vi "S4GUI_001.vi"() -> ()   [LabVIEW 2018] (continued)
                        }
                      }
                    }
                    "Acq status string ch4" <- w721
                    n286 = case shown="True" w726 {
                      tunnel: w729 -> [_ w796]
                      tunnel: w728 -> [_ w799]
                      tunnel: [u32 16739417 w797] -> w727
                      tunnel: ["" ("CamStatus") w796] -> w725
                      frame False {
                      }
                      frame True {
                        n287 = property on="Acq status string ch1" class="Str"() -> ("Text.BGColor"=w798:u32)  [unwired: 2 in, 2 out]
                        n288 = case shown="Default" w796 {
                          tunnel: [w802 u32 13882323 u32 13882323] -> w797
                          tunnel: w799 -> [w801 _ _]
                          tunnel: w798 -> [w800 _ _]
                          frame Default {
                            n289 = case shown="True" w801 {
                              tunnel: [w803 w807] -> w802
                              tunnel: w800 -> [w803 w804]
                              frame False {
                              }
                              frame True {
                                n290 = Equal?(x=w804, y=u32 16776002) -> (x = y?=w806:bool)
                                n291 = case shown="False" w806 {
                                tunnel: [u32 16776002 u32 9346816] -> w807
                                frame False {
                                }
                                frame True {
                                }
                                }
                              }
                            }
                          }
                          frame "IDLE" {
                          }
                          frame "" {
                            # "sem resposta do ACS"
                          }
                        }
                      }
                    }
                    "Acq status string ch1" <- w725
                    n292 = case shown="True" w720 {
                      tunnel: w733 -> [_ w760]
                      tunnel: [u32 16739417 w762] -> w732
                      tunnel: w728 -> [_ w761]
                      tunnel: ["" ("CamStatus") w760] -> w722
                      frame False {
                      }
                      frame True {
                        n293 = property on="Acq status string ch3" class="Str"() -> ("Text.BGColor"=w763:u32)  [unwired: 2 in, 2 out]
                        n294 = case shown="Default" w760 {
                          tunnel: [w766 u32 13882323 u32 13882323] -> w762
                          tunnel: w761 -> [w765 _ _]
                          tunnel: w763 -> [w764 _ _]
                          frame Default {
                            n295 = case shown="True" w765 {
                              tunnel: [w767 w771] -> w766
                              tunnel: w764 -> [w767 w768]
                              frame False {
                              }
                              frame True {
                                n296 = Equal?(x=w768, y=u32 16776002) -> (x = y?=w770:bool)
                                n297 = case shown="True" w770 {
                                tunnel: [u32 16776002 u32 9346816] -> w771
                                frame False {
                                }
                                frame True {
                                }
                                }
                              }
                            }
                          }
                          frame "IDLE" {
                          }
                          frame "" {
                            # "sem resposta do ACS"
                          }
                        }
                      }
                    }
                    "Acq status string ch3" <- w722
                    n298 = case shown="True" w724 {
                      tunnel: w731 -> [_ w778]
                      tunnel: [u32 16739417 w780] -> w730
                      tunnel: w728 -> [_ w779]
                      tunnel: ["" ("CamStatus") w778] -> w723
                      frame False {
                      }
                      frame True {
                        n299 = property on="Acq status string ch2" class="Str"() -> ("Text.BGColor"=w781:u32)  [unwired: 2 in, 2 out]
                        n300 = case shown="\"IDLE\"" w778 {
                          tunnel: [w784 u32 13882323 u32 13882323] -> w780
                          tunnel: w779 -> [w783 _ _]
                          tunnel: w781 -> [w782 _ _]
                          frame Default {
                            n301 = case shown="False" w783 {
                              tunnel: [w785 w789] -> w784
                              tunnel: w782 -> [w785 w786]
                              frame False {
                              }
                              frame True {
                                n302 = Equal?(x=w786, y=u32 16776002) -> (x = y?=w788:bool)
                                n303 = case shown="True" w788 {
                                tunnel: [u32 16776002 u32 9346816] -> w789
                                frame False {
                                }
                                frame True {
                                }
                                }
                              }
                            }
                          }
                          frame "IDLE" {
                          }
                          frame "" {
                            # "sem resposta do ACS"
                          }
                        }
                      }
                    }
                    "Acq status string ch2" <- w723
                    n304 = property on="Acq status string ch2" class="Str"("Text.BGColor"=w730) -> ()  [unwired: 2 in, 2 out]
                    n305 = property on="Acq status string ch1" class="Str"("Text.BGColor"=w727) -> ()  [unwired: 2 in, 2 out]
                    n306 = property on="Acq status string ch3" class="Str"("Text.BGColor"=w732) -> ()  [unwired: 2 in, 2 out]
                    n307 = property on="Acq status string ch4" class="Str"("Text.BGColor"=w735) -> ()  [unwired: 2 in, 2 out]
                  }
                  frame #3 {
                    # "Atualiza status CANAL 1"
                    n308 = Unbundle By Name(w815) -> ("Frames done"=→"Exposure Done ch1":u32, "connection"=→"Channel 1" →"setupCH1":bool, "conf runing"=w812:bool)
                    n309 = property on="setupCH1" class="Bool (strict)"("Blinking"=w812) -> ()  [unwired: 2 in, 2 out]
                  }
                  frame #4 {
                    # "Atualiza status CANAL 2"
                    n310 = Unbundle By Name(w818) -> ("Frames done"=→"Exposure Done ch2":u32, "connection"=→"Channel 2" →"setupCH2":bool, "conf runing"=w816:bool)
                    n311 = property on="setupCH2" class="Bool (strict)"("Blinking"=w816) -> ()  [unwired: 2 in, 2 out]
                  }
                  frame #5 {
                    # "Atualiza status CANAL3"
                    n312 = Unbundle By Name(w822) -> ("Frames done"=→"Exposure Done ch3":u32, "connection"=→"Channel 3" →"setupCH3":bool, "conf runing"=w821:bool)
                    n313 = property on="setupCH3" class="Bool (strict)"("Blinking"=w821) -> ()  [unwired: 2 in, 2 out]
                  }
                  frame #6 {
                    # "Atualiza status CANAL4"
                    n314 = Unbundle By Name(w826) -> ("Frames done"=→"Exposure Done ch4":u32, "connection"=→"Channel 4" →"setupCH4":bool, "conf runing"=w825:bool)
                    n315 = property on="setupCH4" class="Bool (strict)"("Blinking"=w825) -> ()  [unwired: 2 in, 2 out]
                  }
                }
              }
              frame #9 {
                n316 = Unbundle By Name(w829) -> ("Instrument Status.mode"=w828:bool)
                n317 = case shown="True" w828 {
                  tunnel: [0 ("t") w843] -> w830
                  tunnel: w829 -> [_ w832]
                  frame False {
                    # "Fotometria: #PSD = 0"
                  }
                  frame True {
                    # "Polarimetria: calcula #PSD"
                    n318 = Unbundle By Name(w832) -> ("WPROT seq"=w836:u16)
                    n319 = Number To Boolean Array(number=w836) -> (Boolean array=w835:bool[])
                    n320 = for {
                      shift-right: [w847] -> w838
                      shift-left: 0 -> [w845]
                      tunnel: w835 -> [w844] mode=indexing
                      # "calcula qtd de 1s"
                      n321 = Increment(x=w845) -> (x+1=w846:i32)
                      n322 = Select(t=w846, s=w844, f=w845) -> (s? t:f=w847:i32)
                    }
                    n323 = property on="#Polarimetric Sequence Done" class="Slide (strict)"() -> ("Scale.Maximum"=w837:dbl)  [unwired: 2 in, 2 out]
                    n324 = To Long Integer(number=w837) -> (32bit integer=w839:i32)
                    n325 = Subtract(x=w839, y=w838) -> (x-y=w840:i32)
                    n326 = Decrement(x=w840) -> (x-1=w842:i32)
                    n327 = Less Than 0?(x=w842) -> (x < 0?=w841:bool)
                    n328 = Select(t=0, s=w841, f=w842) -> (s? t:f=w843:i32)
                  }
                }
                "#Polarimetric Sequence Done" <- w830
              }
              frame #10 {
                # "OVJ 2022-12-12: \nA visibilidade do Tab ObsEng sempre \nacompanha a habilitação do tab4."
                n329 = Unbundle By Name(w853) -> ("Cluster ExpMode.tab4"=w850:T7, "Cluster Polarimetry"=w874:T15, "Cluster Mode Sync"=w883:T16)
                n330 = case shown="\"Disabled and Grayed Out\"" w850 {
                  tunnel: [TRUE ("Tabs Visible?") w885] -> w852
                  frame "Enabled", Default {
                  }
                  frame "Disabled and Grayed Out" {
                    n331 = disable-structure shown="Enabled" {
                      disable-tunnel: [TRUE ("Tabs Visible?") FALSE ("Tabs Visible?")] -> w885
                      frame Disabled {
                        # "DEBUG"
                      }
                      frame Enabled {
                      }
                    }
                  }
                }
                n332 = property on="Tab ObsEng" class="TabCtl (strict)"("Tabs Visible?"=w852) -> ()  [unwired: 2 in, 2 out]
                n333 = property on="Tab Acq Type" class="TabCtl (strict)"("DisabledEnum"=w850) -> (error out=w851:errorcluster)  [unwired: 2 in, 1 out]
                n334 = Unbundle By Name(w883) -> ("Start SM Text"=w882:string, "Star SM"=w881:T7, "Pause SM"=w880:T7, "Stop SM"=w879:T7, "Abort SM"=w878:T7, "#Cycles"=w877:T7, "SSM"=w876:T7, "Set SM"=w875:T7, "#Index Cycles"=w848:T7)
                n335 = property on="Observer" class="Str"(error in=w851, "DisabledEnum"=w850) -> (error out=w849:errorcluster)  [unwired: 1 in, 1 out]
                n336 = property on="Start SM" class="Bool"("BoolText.Text"=w882) -> ()  [unwired: 2 in, 2 out]
                n337 = property on="set keywords" class="Bool"(error in=w849, "DisabledEnum"=w850) -> ()  [unwired: 1 in, 2 out]
                n338 = property on="#Cycles Done" class="Slide (strict)"("DisabledEnum"=w848) -> ()  [unwired: 2 in, 2 out]
                n339 = property on="Start SM" class="Bool"("DisabledEnum"=w881) -> ()  [unwired: 2 in, 2 out]
                n340 = property on="Stop SM" class="Bool"("DisabledEnum"=w879) -> ()  [unwired: 2 in, 2 out]
                n341 = property on="Abort SM" class="Bool"("DisabledEnum"=w878) -> ()  [unwired: 2 in, 2 out]
                n342 = property on="Pause SM" class="Bool"("DisabledEnum"=w880) -> ()  [unwired: 2 in, 2 out]
                n343 = property on="# Cycles" class="DigNum (strict)"("DisabledEnum"=w877) -> ()  [unwired: 2 in, 2 out]
                n344 = property on="SSM" class="Ring (strict)"("DisabledEnum"=w876) -> ()  [unwired: 2 in, 2 out]
                n345 = property on="Set SM" class="Bool"("DisabledEnum"=w875) -> ()  [unwired: 2 in, 2 out]
                n346 = Unbundle By Name(w874) -> ("Lambda Selector"=w873:T7, "Calibrator Selector"=w872:T7, "Set Waveplate"=w871:T7, "Select Positions"=w870:T7, "P0"=w869:T7, "P8"=w868:T7, "P1"=w867:T7, "P9"=w866:T7, "P2"=w865:T7, "P10"=w864:T7, "P3"=w863:T7, "P11"=w862:T7, "P4"=w861:T7, "P12"=w860:T7, "P5"=w859:T7, "P13"=w858:T7, "P6"=w857:T7, "P14"=w856:T7, "P7"=w855:T7, "P15"=w854:T7)
                n347 = property on="P0" class="Bool (strict)"("DisabledEnum"=w869) -> ()  [unwired: 2 in, 2 out]
                n348 = property on="Lambda Selector" class="Ring (strict)"("DisabledEnum"=w873) -> ()  [unwired: 2 in, 2 out]
                n349 = property on="Calibrator Selector" class="Ring (strict)"("DisabledEnum"=w872) -> ()  [unwired: 2 in, 2 out]
                n350 = property on="Set Waveplate" class="Bool"("DisabledEnum"=w871) -> ()  [unwired: 2 in, 2 out]
                n351 = property on="P1" class="Bool (strict)"("DisabledEnum"=w867) -> ()  [unwired: 2 in, 2 out]
                n352 = property on="P2" class="Bool (strict)"("DisabledEnum"=w865) -> ()  [unwired: 2 in, 2 out]
                n353 = property on="P3" class="Bool (strict)"("DisabledEnum"=w863) -> ()  [unwired: 2 in, 2 out]
                n354 = property on="P4" class="Bool (strict)"("DisabledEnum"=w861) -> ()  [unwired: 2 in, 2 out]
                n355 = property on="P5" class="Bool (strict)"("DisabledEnum"=w859) -> ()  [unwired: 2 in, 2 out]
                n356 = property on="P6" class="Bool (strict)"("DisabledEnum"=w857) -> ()  [unwired: 2 in, 2 out]
                n357 = property on="P7" class="Bool (strict)"("DisabledEnum"=w855) -> ()  [unwired: 2 in, 2 out]
                n358 = property on="Select Positions" class="Ring (strict)"("DisabledEnum"=w870) -> ()  [unwired: 2 in, 2 out]
                n359 = property on="P8" class="Bool (strict)"("DisabledEnum"=w868) -> ()  [unwired: 2 in, 2 out]
                n360 = property on="P15" class="Bool (strict)"("DisabledEnum"=w854) -> ()  [unwired: 2 in, 2 out]
                n361 = property on="P9" class="Bool (strict)"("DisabledEnum"=w866) -> ()  [unwired: 2 in, 2 out]
                n362 = property on="P10" class="Bool (strict)"("DisabledEnum"=w864) -> ()  [unwired: 2 in, 2 out]
                n363 = property on="P11" class="Bool (strict)"("DisabledEnum"=w862) -> ()  [unwired: 2 in, 2 out]
                n364 = property on="P12" class="Bool (strict)"("DisabledEnum"=w860) -> ()  [unwired: 2 in, 2 out]
                n365 = property on="P13" class="Bool (strict)"("DisabledEnum"=w858) -> ()  [unwired: 2 in, 2 out]
                n366 = property on="P14" class="Bool (strict)"("DisabledEnum"=w856) -> ()  [unwired: 2 in, 2 out]
              }
              frame #11 {
                n367 = Unbundle By Name(w902) -> ("Cluster Mode CH1"=w889:T17, "Cluster Mode Sync"=w888:T16)
                n368 = Unbundle By Name(w889) -> ("Start ch1 Text"=w901:string, "#cycles ch1"=w900:T7, "Start ch1"=w899:T7, "Pause ch1"=w898:T7, "Abort ch1"=w897:T7, "Stop ch1"=w896:T7, "Exptime ch1"=w895:T7, "Exp ch1"=w894:T7, "Set Cooler"=w893:T7, "Set Temp"=w892:T7)
                n369 = Unbundle By Name(w888) -> ("#Index Cycles"=w891:T7)
                n370 = case shown="Default" w891 {
                  tunnel: [T7."Enabled" ("#Index Cycles") T7."Disabled and Grayed Out" ("#Index Cycles")] -> w890
                  frame "Disabled and Grayed Out" {
                  }
                  frame Default {
                  }
                }
                n371 = property on="Start ch1" class="Bool"("BoolText.Text"=w901) -> ()  [unwired: 2 in, 2 out]
                n372 = property on="Abort ch1" class="Bool"("DisabledEnum"=w897) -> ()  [unwired: 2 in, 2 out]
                n373 = property on="Stop ch1" class="Bool"("DisabledEnum"=w896) -> ()  [unwired: 2 in, 2 out]
                n374 = property on="#cycles ch1" class="DigNum (strict)"("DisabledEnum"=w900) -> ()  [unwired: 2 in, 2 out]
                n375 = property on="Cooler 1" class="Bool (strict)"("DisabledEnum"=w893) -> ()  [unwired: 2 in, 2 out]
                n376 = property on="Exptime ch1" class="DigNum (strict)"("DisabledEnum"=w895) -> ()  [unwired: 2 in, 2 out]
                n377 = property on="Start ch1" class="Bool"("DisabledEnum"=w899) -> ()  [unwired: 2 in, 2 out]
                n378 = property on="Set Temp 1" class="Bool"("DisabledEnum"=w892) -> ()  [unwired: 2 in, 2 out]
                n379 = property on="Exp ch1" class="DigNum (strict)"("DisabledEnum"=w894) -> ()  [unwired: 2 in, 2 out]
                n380 = property on="Cycles Done ch1" class="Slide (strict)"("DisabledEnum"=w890) -> ()  [unwired: 2 in, 2 out]
                n381 = property on="Pause ch1" class="Bool"("DisabledEnum"=w898) -> ()  [unwired: 2 in, 2 out]
              }
              frame #12 {
                n382 = Unbundle By Name(w919) -> ("Cluster Mode CH2"=w918:T18, "Cluster Mode Sync"=w906:T16)
                n383 = Unbundle By Name(w906) -> ("#Index Cycles"=w907:T7)
                n384 = Unbundle By Name(w918) -> ("Start ch2 Text"=w917:string, "#cycles ch2"=w916:T7, "Start ch2"=w915:T7, "Pause ch2"=w914:T7, "Stop ch2"=w913:T7, "Abort ch2"=w912:T7, "Exptime ch2"=w911:T7, "Exp ch2"=w910:T7, "Set Cooler"=w909:T7, "Set Temp"=w908:T7)
                n385 = case shown="\"Disabled and Grayed Out\"" w907 {
                  tunnel: [T7."Enabled" ("#Index Cycles") T7."Disabled and Grayed Out" ("#Index Cycles")] -> w905
                  frame "Disabled and Grayed Out" {
                  }
                  frame Default {
                  }
                }
                n386 = property on="Start ch2" class="Bool"("BoolText.Text"=w917) -> ()  [unwired: 2 in, 2 out]
                n387 = property on="Stop ch2" class="Bool"("DisabledEnum"=w913) -> ()  [unwired: 2 in, 2 out]
                n388 = property on="Abort ch2" class="Bool"("DisabledEnum"=w912) -> ()  [unwired: 2 in, 2 out]
                n389 = property on="Cooler 2" class="Bool (strict)"("DisabledEnum"=w909) -> ()  [unwired: 2 in, 2 out]
                n390 = property on="#cycles ch2" class="DigNum (strict)"("DisabledEnum"=w916) -> ()  [unwired: 2 in, 2 out]
                n391 = property on="Exptime ch2" class="DigNum (strict)"("DisabledEnum"=w911) -> ()  [unwired: 2 in, 2 out]
                n392 = property on="Set Temp 2" class="Bool"("DisabledEnum"=w908) -> ()  [unwired: 2 in, 2 out]
                n393 = property on="Start ch2" class="Bool"("DisabledEnum"=w915) -> ()  [unwired: 2 in, 2 out]
                n394 = property on="Cycles Done ch2" class="Slide (strict)"("DisabledEnum"=w905) -> ()  [unwired: 2 in, 2 out]
                n395 = property on="Exp ch2" class="DigNum (strict)"("DisabledEnum"=w910) -> ()  [unwired: 2 in, 2 out]
                n396 = property on="Pause ch2" class="Bool"("DisabledEnum"=w914) -> ()  [unwired: 2 in, 2 out]
              }
              frame #13 {
                n397 = Unbundle By Name(w936) -> ("Cluster Mode CH3"=w935:T19, "Cluster Mode Sync"=w923:T16)
                n398 = Unbundle By Name(w923) -> ("#Index Cycles"=w924:T7)
                n399 = Unbundle By Name(w935) -> ("Start ch3 Text"=w934:string, "#cycles ch3"=w933:T7, "Start ch3"=w932:T7, "Pause ch3"=w931:T7, "Stop ch3"=w930:T7, "Abort ch3"=w929:T7, "Exptime ch3"=w928:T7, "Exp ch3"=w927:T7, "Set Cooler"=w926:T7, "Set Temp"=w925:T7)
                n400 = case shown="\"Disabled and Grayed Out\"" w924 {
                  tunnel: [T7."Enabled" ("#Index Cycles") T7."Disabled and Grayed Out" ("#Index Cycles")] -> w922
                  frame "Disabled and Grayed Out" {
                  }
                  frame Default {
                  }
                }
                n401 = property on="Start ch3" class="Bool"("BoolText.Text"=w934) -> ()  [unwired: 2 in, 2 out]
                n402 = property on="Stop ch3" class="Bool"("DisabledEnum"=w930) -> ()  [unwired: 2 in, 2 out]
                n403 = property on="Abort ch3" class="Bool"("DisabledEnum"=w929) -> ()  [unwired: 2 in, 2 out]
                n404 = property on="Cycles Done ch3" class="Slide (strict)"("DisabledEnum"=w922) -> ()  [unwired: 2 in, 2 out]
                n405 = property on="Cooler 3" class="Bool (strict)"("DisabledEnum"=w926) -> ()  [unwired: 2 in, 2 out]
                n406 = property on="#cycles ch3" class="DigNum (strict)"("DisabledEnum"=w933) -> ()  [unwired: 2 in, 2 out]
                n407 = property on="Set Temp 3" class="Bool"("DisabledEnum"=w925) -> ()  [unwired: 2 in, 2 out]
                n408 = property on="Exptime ch3" class="DigNum (strict)"("DisabledEnum"=w928) -> ()  [unwired: 2 in, 2 out]
                n409 = property on="Start ch3" class="Bool"("DisabledEnum"=w932) -> ()  [unwired: 2 in, 2 out]
                n410 = property on="Exp ch3" class="DigNum (strict)"("DisabledEnum"=w927) -> ()  [unwired: 2 in, 2 out]
                n411 = property on="Pause ch3" class="Bool"("DisabledEnum"=w931) -> ()  [unwired: 2 in, 2 out]
              }
              frame #14 {
                n412 = Unbundle By Name(w953) -> ("Cluster Mode CH4"=w952:T20, "Cluster Mode Sync"=w940:T16)
                n413 = Unbundle By Name(w940) -> ("#Index Cycles"=w941:T7)
                n414 = Unbundle By Name(w952) -> ("Start ch4 Text"=w951:string, "#cycles ch4"=w950:T7, "Start ch4"=w949:T7, "Pause ch4"=w948:T7, "Stop ch4"=w947:T7, "Abort ch4"=w946:T7, "Exptime ch4"=w945:T7, "Exp ch4"=w944:T7, "Set Cooler"=w943:T7, "Set Temp"=w942:T7)
                n415 = case shown="\"Disabled and Grayed Out\"" w941 {
                  tunnel: [T7."Enabled" ("#Index Cycles") T7."Disabled and Grayed Out" ("#Index Cycles")] -> w939
                  frame "Disabled and Grayed Out" {
                  }
                  frame Default {
                  }
                }
                n416 = property on="Start ch4" class="Bool"("BoolText.Text"=w951) -> ()  [unwired: 2 in, 2 out]
                n417 = property on="Stop ch4" class="Bool"("DisabledEnum"=w947) -> ()  [unwired: 2 in, 2 out]
                n418 = property on="Cooler 4" class="Bool (strict)"("DisabledEnum"=w943) -> ()  [unwired: 2 in, 2 out]
                n419 = property on="Set Temp 4" class="Bool"("DisabledEnum"=w942) -> ()  [unwired: 2 in, 2 out]
                n420 = property on="Abort ch4" class="Bool"("DisabledEnum"=w946) -> ()  [unwired: 2 in, 2 out]
                n421 = property on="#cycles ch4" class="DigNum (strict)"("DisabledEnum"=w950) -> ()  [unwired: 2 in, 2 out]
                n422 = property on="Exptime ch4" class="DigNum (strict)"("DisabledEnum"=w945) -> ()  [unwired: 2 in, 2 out]
                n423 = property on="Cycles Done ch4" class="Slide (strict)"("DisabledEnum"=w939) -> ()  [unwired: 2 in, 2 out]
                n424 = property on="Start ch4" class="Bool"("DisabledEnum"=w949) -> ()  [unwired: 2 in, 2 out]
                n425 = property on="Exp ch4" class="DigNum (strict)"("DisabledEnum"=w944) -> ()  [unwired: 2 in, 2 out]
                n426 = property on="Pause ch4" class="Bool"("DisabledEnum"=w948) -> ()  [unwired: 2 in, 2 out]
              }
              frame #15 {
                # "Carrega coluna do Channel 1"
                # "Aba:  Eng->Camera"
                n427 = Unbundle By Name(w1039) -> ("ChannelA_CCD"=w963:T21, "CHA_Checked Params"=w1030:T22, "ChannelA_Status.connection"=w962:bool)
                n428 = Unbundle By Name(w1030) -> ("ACQUISITION_MODE"=w987:bool, "TRIGGER_MODE"=w988:bool, "READ_MODE"=w989:bool, "PREAMP"=w997:bool, "READOUT_RATE"=w998:bool, "VERTICAL_SHIFT_SPEED"=w999:bool, "EM_MODE"=w1000:bool, "EM_GAIN"=w990:bool, "SHUTTER_MODE"=w991:bool, "SHUTTER_TTL"=w992:bool, "SHUTTER_OPENING_TIME"=w993:bool, "SHUTTER_CLOSING_TIME"=w994:bool, "VBIN"=w995:bool, "HBIN"=w996:bool, "INITIAL_LINE"=w1008:bool, "INITIAL_COLUMN"=w1024:bool, "FINAL_LINE"=w1029:bool, "FINAL_COLUMN"=w1022:bool, "FRAME_TRANSFER"=w1018:bool, "VERTICAL_CLOCK_VOLTAGE"=w1017:bool, "AD_CHANNEL"=w1016:bool)
                n429 = Unbundle By Name(w963) -> ("INITIAL_LINE"=w985:u16, "INITIAL_COLUMN"=w984:u16, "FINAL_LINE"=w983:u16, "FINAL_COLUMN"=w982:u16, "VBIN"=w981:u16, "HBIN"=w980:u16, "PREAMP"=w979:u8, "EM_GAIN"=w978:u16, "READOUT_RATE"=w977:u8, "SHUTTER_OPENNING_TIME"=w976:u16, "SHUTTER_CLOSING_TIME"=w975:u16, "VERTICAL_SHIFT_SPEED"=w974:u8, "READ_MODE"=w973:u8, "VERTICAL_CLOCK_VOLTAGE"=w972:u8, "AD_CHANNEL"=w971:u32, "SHUTTER_MODE"=w970:u8, "SHUTTER_TTL"=w969:u8, "TRIGGER_MODE"=w968:u8, "FRAME_TRANSFER"=w967:bool, "ACQUISITION_MODE"=w965:u8, "EM_MODE"=w964:u8)
                n430 = Equal?(x=w1034, y="none") -> (x = y?=w1031:bool)
                n431 = Equal?(x=w1034, y="default.cfg") -> (x = y?=w1032:bool)
                n432 = Or(x=w1032, y=w1031) -> (x .or. y?=w1033:bool)
                n433 = case shown="True" w1033 {
                  tunnel: [T7."Enabled" ("Disabled") T7."Disabled and Grayed Out" ("Disabled")] -> w1036
                  frame False {
                    # "Se Curr Conf File != default.cfg,\nhabilita botão de Salvar."
                  }
                  frame True {
                    # "Não é permitido salvar em \ncima de default.cfg"
                  }
                }
                n434 = case shown="True" w962 {
                  tunnel: w963 -> [_ w1047]
                  tunnel: [w1040 w1046] -> w961
                  tunnel: [w1040 w1045] -> w960
                  tunnel: [w1040 w1044] -> w959
                  tunnel: [w1040 w1043] -> w958
                  tunnel: [w1040 w1042] -> w957
                  tunnel: [w1040 w1041] -> w956
                  frame False {
                    w1040 = "" ("RO1")
                  }
                  frame True {
                    n435 = stacked-sequence "Atualizacao dos indicadores inferiores do CANAL A da tela principal" {
                      tunnel: w1047 -> [w1062 w1065 w1070 w1079 w1082 w1086]
                      tunnel: [w1048 _ _ _ _ _] -> w1046
                      tunnel: [_ w1063 _ _ _ _] -> w1045
                      tunnel: [_ _ w1068 _ _ _] -> w1044
                      tunnel: [_ _ _ w1073 _ _] -> w1043
                      tunnel: [_ _ _ _ w1080 _] -> w1042
                      tunnel: [_ _ _ _ _ w1083] -> w1041
                      frame #0 {
                        # "SubImage"
                        n436 = Unbundle By Name(w1062) -> ("INITIAL_LINE"=w1060:u16, "FINAL_LINE"=w1059:u16, "INITIAL_COLUMN"=w1058:u16, "FINAL_COLUMN"=w1057:u16)
                        n437 = Number To Decimal String(number=w1060) -> (decimal integer string=w1056:string)  [unwired: 1 in]
                        n438 = Number To Decimal String(number=w1059) -> (decimal integer string=w1054:string)  [unwired: 1 in]
                        n439 = Number To Decimal String(number=w1058) -> (decimal integer string=w1052:string)  [unwired: 1 in]
                        n440 = Number To Decimal String(number=w1057) -> (decimal integer string=w1050:string)  [unwired: 1 in]
                        n441 = Concatenate Strings("[", w1056, ":", w1054, ",", w1052, ":", w1050, "]") -> (w1048:string)
                      }
                      frame #1 {
                        # "Em Active"
                        n442 = Unbundle By Name(w1065) -> ("EM_MODE"=w1064:u8)
                        n443 = case shown="0, Default" w1064 {
                          tunnel: ["Electron M." ("EmActive1") "Convent." ("EmActive1")] -> w1063
                          frame 0, Default {
                          }
                          frame 1 {
                          }
                        }
                      }
                      frame #2 {
                        # "Pre Amp"
                        n444 = Unbundle By Name(w1070) -> ("PREAMP"=w1069:u8)
                        n445 = case shown="1" w1069 {
                          tunnel: ["Gain 1" ("EmActive1") "Gain 2" ("EmActive1")] -> w1068
                          frame 0, Default {
                          }
                          frame 1 {
                          }
                        }
                      }
                      frame #3 {
                        # "Binning"
                        n446 = Unbundle By Name(w1079) -> ("VBIN"=w1078:u16, "HBIN"=w1077:u16)
                        n447 = Number To Decimal String(number=w1077) -> (decimal integer string=w1074:string)  [unwired: 1 in]
                        n448 = Number To Decimal String(number=w1078) -> (decimal integer string=w1076:string)  [unwired: 1 in]
                        n449 = Concatenate Strings(w1076, "x", w1074) -> (w1073:string)
                      }
                      frame #4 {
                        # "Gain"
                        n450 = Unbundle By Name(w1082) -> ("EM_GAIN"=w1081:u16)
                        n451 = Number To Decimal String(number=w1081) -> (decimal integer string=w1080:string)  [unwired: 1 in]
                      }
                      frame #5 {
                        # "Readout"
                        n452 = Unbundle By Name(w1086) -> ("EM_MODE"=w1085:u8, "READOUT_RATE"=w1084:u8)
                        n453 = case shown="1" w1085 {
                          tunnel: w1084 -> [w1088 w1094]
                          tunnel: [w1087 w1093] -> w1083
                          frame 0, Default {
                            n454 = case shown="3" w1088 {
                              tunnel: ["30 MHz" ("EmActive1") "20 MHz" ("EmActive1") "10 MHz" ("EmActive1") "1 MHz" ("EmActive1")] -> w1087
                              frame 0, Default {
                              }
                              frame 1 {
                              }
                              frame 2 {
                              }
                              frame 3 {
                              }
                            }
                          }
                          frame 1 {
                            n455 = case shown="1" w1094 {
                              tunnel: ["1 MHz" ("EmActive1") "0.1 MHz" ("EmActive1")] -> w1093
                              frame 0, Default {
                              }
                              frame 1 {
                              }
                            }
                          }
                        }
                      }
                    }
                  }
                }
                n456 = Not(x=w1022) -> (.not. x?=w1023:bool)
                n457 = Not(x=w1018) -> (.not. x?=w1020:bool)
                n458 = Not(x=w1017) -> (.not. x?=w1021:bool)
                n459 = Not(x=w1016) -> (.not. x?=w1019:bool)
                n460 = Not(x=w1008) -> (.not. x?=w1026:bool)
                n461 = Not(x=w1024) -> (.not. x?=w1025:bool)
                n462 = Not(x=w1029) -> (.not. x?=w1028:bool)
                n463 = property on="Image FInal Column" class="DigNum (strict)"("Blinking"=w1023) -> ()  [unwired: 2 in, 2 out]
                n464 = property on="Frame Transfer" class="Bool (strict)"("Blinking"=w1020) -> ()  [unwired: 2 in, 2 out]
                n465 = property on="Vertical Clock Voltage" class="Ring (strict)"("Blinking"=w1021) -> ()  [unwired: 2 in, 2 out]
                n466 = property on="A/D  Channel" class="DigNum (strict)"("Blinking"=w1019) -> ()  [unwired: 2 in, 2 out]
                n467 = property on="Image Initial Line" class="DigNum (strict)"("Blinking"=w1026) -> ()  [unwired: 2 in, 2 out]
                n468 = property on="Image Initial Column" class="DigNum (strict)"("Blinking"=w1025) -> ()  [unwired: 2 in, 2 out]
                n469 = property on="Image Final Line" class="DigNum (strict)"("Blinking"=w1028) -> ()  [unwired: 2 in, 2 out]
                n470 = property on="Save Button" class="Bool (strict)"("DisabledEnum"=w1036) -> ()  [unwired: 2 in, 2 out]
                n471 = Not(x=w993) -> (.not. x?=w1012:bool)
                n472 = Not(x=w994) -> (.not. x?=w1014:bool)
                n473 = Not(x=w995) -> (.not. x?=w1013:bool)
                n474 = Not(x=w996) -> (.not. x?=w1015:bool)
                n475 = Not(x=w990) -> (.not. x?=w1010:bool)
                n476 = Not(x=w991) -> (.not. x?=w1011:bool)
                n477 = Not(x=w992) -> (.not. x?=w1009:bool)
                n478 = property on="Shutter Openning Time" class="DigNum (strict)"("Blinking"=w1012) -> ()  [unwired: 2 in, 2 out]
                n479 = property on="Shutter Closing Time" class="DigNum (strict)"("Blinking"=w1014) -> ()  [unwired: 2 in, 2 out]
                n480 = property on="Vertical Binning" class="DigNum (strict)"("Blinking"=w1013) -> ()  [unwired: 2 in, 2 out]
                n481 = property on="Horizontal Binning" class="DigNum (strict)"("Blinking"=w1015) -> ()  [unwired: 2 in, 2 out]
                n482 = property on="CCD EM Gain" class="DigNum (strict)"("Blinking"=w1010) -> ()  [unwired: 2 in, 2 out]
                n483 = property on="Shutter Mode" class="Ring (strict)"("Blinking"=w1011) -> ()  [unwired: 2 in, 2 out]
                n484 = property on="Shutter TTL" class="Ring (strict)"("Blinking"=w1009) -> ()  [unwired: 2 in, 2 out]
                n485 = First Call?() -> (First Call?: T/F=w986:bool)
                n486 = case shown="True" w986 {
                  tunnel: w985 -> [_ w1117]
                  tunnel: w984 -> [_ w1116]
                  tunnel: w983 -> [_ w1115]
                  tunnel: w982 -> [_ w1114]
                  tunnel: w981 -> [_ w1113]
                  tunnel: w980 -> [_ w1112]
                  tunnel: w979 -> [_ w1111]
                  tunnel: w978 -> [_ w1110]
                  tunnel: w977 -> [_ w1109]
                  tunnel: w976 -> [_ w1108]
                  tunnel: w975 -> [_ w1107]
                  tunnel: w974 -> [_ w1106]
                  tunnel: w973 -> [_ w1105]
                  tunnel: w972 -> [_ w1104]
                  tunnel: w971 -> [_ w1103]
                  tunnel: w970 -> [_ w1102]
                  tunnel: w969 -> [_ w1101]
                  tunnel: w968 -> [_ w1100]
                  tunnel: w967 -> [_ w1099]
                  tunnel: w965 -> [_ w1098]
                  tunnel: w964 -> [_ w1097]
                  frame False {
                  }
                  frame True {
                    n487 = local read "Input Cluster"() -> (w1121:T6)
                    n488 = Unbundle By Name(w1121) -> ("Parameters"=w1119:T23)
                    n489 = Bundle By Name(cluster=w1119, "Image \nInitial Line"=w1117, "Image\nInitial Column"=w1116, "Image\nFinal Line"=w1115, "Image\nFInal Column"=w1114, "Vertical\nBinning"=w1113, "Horizontal\nBinning"=w1112, "Pre-amplification\nGain"=w1111, "CCD\nEM Gain"=w1110, "Readout\nRate"=w1109, "Shutter\nOpenning Time"=w1108, "Shutter\nClosing Time"=w1107, "Vertical\nShift Speed"=w1106, "Read\nMode"=w1105, "Vertical\nClock Voltage"=w1104, "A/D \nChannel"=w1103, "Shutter\nMode"=w1102, "Shutter\nTTL"=w1101, "Trigger\nMode"=w1100, "Frame\nTransfer"=w1099, "Acquisition\nMode"=w1098, "CCD \nEM Mode"=w1097) -> (w1118:T23)
                    n490 = Bundle By Name(cluster=w1121, "Parameters"=w1118) -> (w1120:T6)
                    n491 = local write "Input Cluster"(w1120) -> ()
                  }
                }
                n492 = Not(x=w987) -> (.not. x?=w1001:bool)
                n493 = local read "Cameras Cluster"() -> (w1038:T5)
                n494 = Bundle By Name(cluster=w1038, "Current Configuration.Image Initial Line"=w985, "Current Configuration.Image Initial Column"=w984, "Current Configuration.Image Final Line"=w983, "Current Configuration.Image FInal Column"=w982, "Current Configuration.Vertical Binning"=w981, "Current Configuration.Horizontal Binning"=w980, "Current Configuration.Pre-amplification Gain"=w979, "Current Configuration.CCD EM Gain"=w978, "Current Configuration.Readout Rate"=w977, "Current Configuration.Shutter Openning Time"=w976, "Current Configuration.Shutter Closing Time"=w975, "Current Configuration.Vertical Shift Speed"=w974, "Current Configuration.Read Mode"=w973, "Current Configuration.Vertical Clock Voltage"=w972, "Current Configuration.A/D  Channel"=w971, "Current Configuration.Shutter Mode"=w970, "Current Configuration.Shutter TTL"=w969, "Current Configuration.Trigger Mode"=w968, "Current Configuration.Frame Transfer"=w967, "Current Configuration.Acquisition Mode"=w965, "Current Configuration.CCD EM Mode"=w964) -> (w966:T5)
                n495 = Not(x=w998) -> (.not. x?=w1004:bool)
                n496 = Not(x=w999) -> (.not. x?=w1002:bool)
                n497 = Not(x=w1000) -> (.not. x?=w1003:bool)
                n498 = Not(x=w988) -> (.not. x?=w1006:bool)
                n499 = Not(x=w989) -> (.not. x?=w1005:bool)
                n500 = Not(x=w997) -> (.not. x?=w1007:bool)
                n501 = local write "RO1"(w956) -> ()
                n502 = local write "SI1"(w961) -> ()
                n503 = local write "EA1"(w960) -> ()
                n504 = local write "PA1"(w959) -> ()
                n505 = local write "B1"(w958) -> ()
                n506 = local write "G1"(w957) -> ()
                n507 = property on="Acquisition Mode" class="Ring (strict)"("Blinking"=w1001) -> ()  [unwired: 2 in, 2 out]
                n508 = property on="Readout Rate" class="Ring (strict)"("Blinking"=w1004) -> ()  [unwired: 2 in, 2 out]
                n509 = property on="Vertical Shift Speed" class="Ring (strict)"("Blinking"=w1002) -> ()  [unwired: 2 in, 2 out]
                n510 = property on="CCD EM Mode" class="Ring (strict)"("Blinking"=w1003) -> ()  [unwired: 2 in, 2 out]
                n511 = property on="Trigger Mode" class="Ring (strict)"("Blinking"=w1006) -> ()  [unwired: 2 in, 2 out]
                n512 = property on="Read Mode" class="Ring (strict)"("Blinking"=w1005) -> ()  [unwired: 2 in, 2 out]
                n513 = property on="Pre-amplification Gain" class="Ring (strict)"("Blinking"=w1007) -> ()  [unwired: 2 in, 2 out]
                n514 = local write "Cameras Cluster"(w966) -> ()
                n515 = Compound Arithmetic op=AND(w987, w988, w989, w997, w998, w999, w1000, w990, w991, w992, w993, w994, w995, w996, w1008, w1024, w1029, w1022, w1018, w1017, w1016) -> (→"CCD checked 1":bool)
                "Current Configuration File:" <- w1034
              }
              frame #16 {
                # "Carrega coluna do Channel 2"
                # "Aba:  Eng->Camera"
                n516 = Unbundle By Name(w1199) -> ("ChannelB_CCD"=w1131:T21, "CHB_Checked Params"=w1132:T22, "ChannelB_Status.connection"=w1130:bool)
                n517 = Unbundle By Name(w1132) -> ("ACQUISITION_MODE"=w1150:bool, "TRIGGER_MODE"=w1149:bool, "READ_MODE"=w1148:bool, "PREAMP"=w1147:bool, "READOUT_RATE"=w1146:bool, "VERTICAL_SHIFT_SPEED"=w1145:bool, "EM_MODE"=w1144:bool, "EM_GAIN"=w1157:bool, "SHUTTER_MODE"=w1156:bool, "SHUTTER_TTL"=w1155:bool, "SHUTTER_OPENING_TIME"=w1154:bool, "SHUTTER_CLOSING_TIME"=w1153:bool, "VBIN"=w1152:bool, "HBIN"=w1151:bool, "INITIAL_LINE"=w1164:bool, "INITIAL_COLUMN"=w1163:bool, "FINAL_LINE"=w1162:bool, "FINAL_COLUMN"=w1161:bool, "FRAME_TRANSFER"=w1160:bool, "VERTICAL_CLOCK_VOLTAGE"=w1159:bool, "AD_CHANNEL"=w1158:bool)
                n518 = case shown="True" w1130 {
                  tunnel: w1131 -> [_ w1207]
                  tunnel: [w1200 w1206] -> w1129
                  tunnel: [w1200 w1205] -> w1128
                  tunnel: [w1200 w1204] -> w1127
                  tunnel: [w1200 w1203] -> w1126
                  tunnel: [w1200 w1202] -> w1125
                  tunnel: [w1200 w1201] -> w1124
                  frame False {
                    w1200 = "" ("EmActive1")
                  }
                  frame True {
                    n519 = stacked-sequence "Atualizacao dos indicadores inferiores do CANAL B da tela principal" {
                      tunnel: w1207 -> [w1222 w1225 w1230 w1239 w1242 w1246]
                      tunnel: [_ w1223 _ _ _ _] -> w1206
                      tunnel: [_ _ w1228 _ _ _] -> w1205
                      tunnel: [_ _ _ w1233 _ _] -> w1204
                      tunnel: [_ _ _ _ w1240 _] -> w1203
                      tunnel: [_ _ _ _ _ w1243] -> w1202
                      tunnel: [w1208 _ _ _ _ _] -> w1201
                      frame #0 {
                        # "SubImage"
                        n520 = Unbundle By Name(w1222) -> ("INITIAL_LINE"=w1220:u16, "FINAL_LINE"=w1219:u16, "INITIAL_COLUMN"=w1218:u16, "FINAL_COLUMN"=w1217:u16)
                        n521 = Number To Decimal String(number=w1220) -> (decimal integer string=w1216:string)  [unwired: 1 in]
                        n522 = Number To Decimal String(number=w1219) -> (decimal integer string=w1214:string)  [unwired: 1 in]
                        n523 = Number To Decimal String(number=w1218) -> (decimal integer string=w1212:string)  [unwired: 1 in]
                        n524 = Number To Decimal String(number=w1217) -> (decimal integer string=w1210:string)  [unwired: 1 in]
                        n525 = Concatenate Strings("[", w1216, ":", w1214, ",", w1212, ":", w1210, "]") -> (w1208:string)
                      }
                      frame #1 {
                        # "Em Active"
                        n526 = Unbundle By Name(w1225) -> ("EM_MODE"=w1224:u8)
                        n527 = case shown="0, Default" w1224 {
                          tunnel: ["Electron M." ("EmActive1") "Convent." ("EmActive1")] -> w1223
                          frame 0, Default {
                          }
                          frame 1 {
                          }
                        }
                      }
                      frame #2 {
                        # "Pre Amp"
                        n528 = Unbundle By Name(w1230) -> ("PREAMP"=w1229:u8)
                        n529 = case shown="1" w1229 {
                          tunnel: ["Gain 1" ("EmActive1") "Gain 2" ("EmActive1")] -> w1228
                          frame 0, Default {
                          }
                          frame 1 {
                          }
                        }
                      }
                      frame #3 {
                        # "Binning"
                        n530 = Unbundle By Name(w1239) -> ("VBIN"=w1238:u16, "HBIN"=w1237:u16)
                        n531 = Number To Decimal String(number=w1237) -> (decimal integer string=w1235:string)  [unwired: 1 in]
                        n532 = Number To Decimal String(number=w1238) -> (decimal integer string=w1236:string)  [unwired: 1 in]
                        n533 = Concatenate Strings(w1236, "x", w1235) -> (w1233:string)
                      }
                      frame #4 {
                        # "Gain"
                        n534 = Unbundle By Name(w1242) -> ("EM_GAIN"=w1241:u16)
                        n535 = Number To Decimal String(number=w1241) -> (decimal integer string=w1240:string)  [unwired: 1 in]
                      }
                      frame #5 {
                        # "Readout"
                        n536 = Unbundle By Name(w1246) -> ("EM_MODE"=w1245:u8, "READOUT_RATE"=w1244:u8)
                        n537 = case shown="0, Default" w1245 {
                          tunnel: w1244 -> [w1248 w1254]
                          tunnel: [w1247 w1253] -> w1243
                          frame 0, Default {
                            n538 = case shown="0, Default" w1248 {
                              tunnel: ["30 MHz" ("EmActive1") "20 MHz" ("EmActive1") "10 MHz" ("EmActive1") "1 MHz" ("EmActive1")] -> w1247
                              frame 0, Default {
                              }
                              frame 1 {
                              }
                              frame 2 {
                              }
                              frame 3 {
                              }
                            }
                          }
                          frame 1 {
                            n539 = case shown="1" w1254 {
                              tunnel: ["1 MHz" ("EmActive1") "0.1 MHz" ("EmActive1")] -> w1253
                              frame 0, Default {
                              }
                              frame 1 {
                              }
                            }
                          }
                        }
                      }
                    }
                  }
                }
                n540 = Unbundle By Name(w1131) -> ("INITIAL_LINE"=w1137:u16, "INITIAL_COLUMN"=w1135:u16, "FINAL_LINE"=w1138:u16, "FINAL_COLUMN"=w1136:u16, "VBIN"=w1141:u16, "HBIN"=w1196:u16, "PREAMP"=w1140:u8, "EM_GAIN"=w1139:u16, "READOUT_RATE"=w1134:u8, "SHUTTER_OPENNING_TIME"=w1195:u16, "SHUTTER_CLOSING_TIME"=w1194:u16, "VERTICAL_SHIFT_SPEED"=w1193:u8, "READ_MODE"=w1192:u8, "VERTICAL_CLOCK_VOLTAGE"=w1191:u8, "AD_CHANNEL"=w1190:u32, "SHUTTER_MODE"=w1187:u8, "SHUTTER_TTL"=w1188:u8, "TRIGGER_MODE"=w1142:u8, "FRAME_TRANSFER"=w1143:bool, "ACQUISITION_MODE"=w1189:u8, "EM_MODE"=w1133:u8)
                n541 = Not(x=w1161) -> (.not. x?=w1182:bool)
                n542 = Not(x=w1160) -> (.not. x?=w1180:bool)
                n543 = Not(x=w1159) -> (.not. x?=w1181:bool)
                n544 = Not(x=w1158) -> (.not. x?=w1179:bool)
                n545 = Not(x=w1164) -> (.not. x?=w1184:bool)
                n546 = Not(x=w1163) -> (.not. x?=w1183:bool)
                n547 = Not(x=w1162) -> (.not. x?=w1185:bool)
                n548 = property on="Image FInal Column 2" class="DigNum (strict)"("Blinking"=w1182) -> ()  [unwired: 2 in, 2 out]
                n549 = property on="Frame Transfer 2" class="Bool (strict)"("Blinking"=w1180) -> ()  [unwired: 2 in, 2 out]
                n550 = property on="Vertical Clock Voltage 2" class="Ring (strict)"("Blinking"=w1181) -> ()  [unwired: 2 in, 2 out]
                n551 = property on="A/D Channel 2" class="DigNum (strict)"("Blinking"=w1179) -> ()  [unwired: 2 in, 2 out]
                n552 = property on="Image Initial Line 2" class="DigNum (strict)"("Blinking"=w1184) -> ()  [unwired: 2 in, 2 out]
                n553 = property on="Image Initial Column 2" class="DigNum (strict)"("Blinking"=w1183) -> ()  [unwired: 2 in, 2 out]
                n554 = property on="Image Final Line 2" class="DigNum (strict)"("Blinking"=w1185) -> ()  [unwired: 2 in, 2 out]
                n555 = Not(x=w1154) -> (.not. x?=w1175:bool)
                n556 = Not(x=w1153) -> (.not. x?=w1177:bool)
                n557 = Not(x=w1152) -> (.not. x?=w1176:bool)
                n558 = Not(x=w1151) -> (.not. x?=w1178:bool)
                n559 = Not(x=w1157) -> (.not. x?=w1173:bool)
                n560 = Not(x=w1156) -> (.not. x?=w1174:bool)
                n561 = Not(x=w1155) -> (.not. x?=w1172:bool)
                n562 = property on="Shutter Openning Time 2" class="DigNum (strict)"("Blinking"=w1175) -> ()  [unwired: 2 in, 2 out]
                n563 = property on="Shutter Closing Time 2" class="DigNum (strict)"("Blinking"=w1177) -> ()  [unwired: 2 in, 2 out]
                n564 = property on="Vertical Binning 2" class="DigNum (strict)"("Blinking"=w1176) -> ()  [unwired: 2 in, 2 out]
                n565 = property on="Horizontal Binning 2" class="DigNum (strict)"("Blinking"=w1178) -> ()  [unwired: 2 in, 2 out]
                n566 = property on="CCD EM Gain 2" class="DigNum (strict)"("Blinking"=w1173) -> ()  [unwired: 2 in, 2 out]
                n567 = property on="Shutter Mode 2" class="Ring (strict)"("Blinking"=w1174) -> ()  [unwired: 2 in, 2 out]
                n568 = property on="Shutter TTL 2" class="Ring (strict)"("Blinking"=w1172) -> ()  [unwired: 2 in, 2 out]
                n569 = local read "Cameras Cluster"() -> (w1198:T5)
                n570 = Bundle By Name(cluster=w1198, "Current Configuration.Image Initial Line 2"=w1137, "Current Configuration.Image Initial Column 2"=w1135, "Current Configuration.Image Final Line 2"=w1138, "Current Configuration.Image FInal Column 2"=w1136, "Current Configuration.Vertical Binning 2"=w1141, "Current Configuration.Horizontal Binning 2"=w1196, "Current Configuration.Pre-amplification Gain 2"=w1140, "Current Configuration.CCD EM Gain 2"=w1139, "Current Configuration.Readout Rate 2"=w1134, "Current Configuration.Shutter Openning Time 2"=w1195, "Current Configuration.Shutter Closing Time 2"=w1194, "Current Configuration.Vertical Shift Speed 2"=w1193, "Current Configuration.Read Mode 2"=w1192, "Current Configuration.Vertical Clock Voltage 2"=w1191, "Current Configuration.A/D Channel 2"=w1190, "Current Configuration.Shutter Mode 2"=w1187, "Current Configuration.Shutter TTL 2"=w1188, "Current Configuration.Trigger Mode 2"=w1142, "Current Configuration.Frame Transfer 2"=w1143, "Current Configuration.Acquisition Mode 2"=w1189, "Current Configuration.CCD EM Mode 2"=w1133) -> (w1197:T5)
                n571 = local write "PA2"(w1128) -> ()
                n572 = local write "B2"(w1127) -> ()
                n573 = local write "EA2"(w1129) -> ()
                n574 = local write "SI2"(w1124) -> ()
                n575 = local write "RO2"(w1125) -> ()
                n576 = local write "G2"(w1126) -> ()
                n577 = Not(x=w1150) -> (.not. x?=w1165:bool)
                n578 = Not(x=w1146) -> (.not. x?=w1168:bool)
                n579 = Not(x=w1145) -> (.not. x?=w1166:bool)
                n580 = Not(x=w1144) -> (.not. x?=w1167:bool)
                n581 = Not(x=w1149) -> (.not. x?=w1170:bool)
                n582 = Not(x=w1148) -> (.not. x?=w1169:bool)
                n583 = Not(x=w1147) -> (.not. x?=w1171:bool)
                n584 = property on="Acquisition Mode 2" class="Ring (strict)"("Blinking"=w1165) -> ()  [unwired: 2 in, 2 out]
                n585 = property on="Readout Rate 2" class="Ring (strict)"("Blinking"=w1168) -> ()  [unwired: 2 in, 2 out]
                n586 = property on="Vertical Shift Speed 2" class="Ring (strict)"("Blinking"=w1166) -> ()  [unwired: 2 in, 2 out]
                n587 = property on="CCD EM Mode 2" class="Ring (strict)"("Blinking"=w1167) -> ()  [unwired: 2 in, 2 out]
                n588 = property on="Trigger Mode 2" class="Ring (strict)"("Blinking"=w1170) -> ()  [unwired: 2 in, 2 out]
                n589 = property on="Read Mode 2" class="Ring (strict)"("Blinking"=w1169) -> ()  [unwired: 2 in, 2 out]
                n590 = property on="Pre-amplification Gain 2" class="Ring (strict)"("Blinking"=w1171) -> ()  [unwired: 2 in, 2 out]
                n591 = local write "Cameras Cluster"(w1197) -> ()
                n592 = Compound Arithmetic op=AND(w1150, w1149, w1148, w1147, w1146, w1145, w1144, w1157, w1156, w1155, w1154, w1153, w1152, w1151, w1164, w1163, w1162, w1161, w1160, w1159, w1158) -> (→"CCD checked 2":bool)
              }
              frame #17 {
                # "Carrega coluna do Channel 3"
                # "Aba:  Eng->Camera"
                n593 = Unbundle By Name(w1332) -> ("ChannelC_CCD"=w1264:T21, "CHC_Checked Params"=w1317:T22, "ChannelC_Status.connection"=w1257:bool)
                n594 = Unbundle By Name(w1317) -> ("ACQUISITION_MODE"=w1280:bool, "TRIGGER_MODE"=w1279:bool, "READ_MODE"=w1278:bool, "PREAMP"=w1277:bool, "READOUT_RATE"=w1276:bool, "VERTICAL_SHIFT_SPEED"=w1275:bool, "EM_MODE"=w1274:bool, "EM_GAIN"=w1288:bool, "SHUTTER_MODE"=w1287:bool, "SHUTTER_TTL"=w1285:bool, "SHUTTER_OPENING_TIME"=w1284:bool, "SHUTTER_CLOSING_TIME"=w1283:bool, "VBIN"=w1282:bool, "HBIN"=w1281:bool, "INITIAL_LINE"=w1295:bool, "INITIAL_COLUMN"=w1294:bool, "FINAL_LINE"=w1293:bool, "FINAL_COLUMN"=w1292:bool, "FRAME_TRANSFER"=w1291:bool, "VERTICAL_CLOCK_VOLTAGE"=w1290:bool, "AD_CHANNEL"=w1289:bool)
                n595 = case shown="True" w1257 {
                  tunnel: w1264 -> [_ w1340]
                  tunnel: [w1333 w1339] -> w1263
                  tunnel: [w1333 w1338] -> w1262
                  tunnel: [w1333 w1337] -> w1261
                  tunnel: [w1333 w1336] -> w1260
                  tunnel: [w1333 w1335] -> w1259
                  tunnel: [w1333 w1334] -> w1258
                  frame False {
                    w1333 = ""
                  }
                  frame True {
